vi "Configure Trace Statistics.vi"(7 "User Domain (0)":dbl, 8 "error in (no error)":errorcluster, 9 "Statistic Type (0: Peak to Peak)":i32(ring) items=["Peak to Peak", "Standard Deviation", "Mean", "Min", "Max"], 10 "Channel (1)":i32=1, 11 "VISA resource name":refnum<visa-resource-name>) -> (0 "error out":errorcluster, 3 "VISA resource name out":refnum<visa-resource-name>)   [LabVIEW 2018, in "Keysight PNA Series.lvlib"]
doc: "Configure Trace Statistics."
uses:
  Keysight PNA Series.lvlib
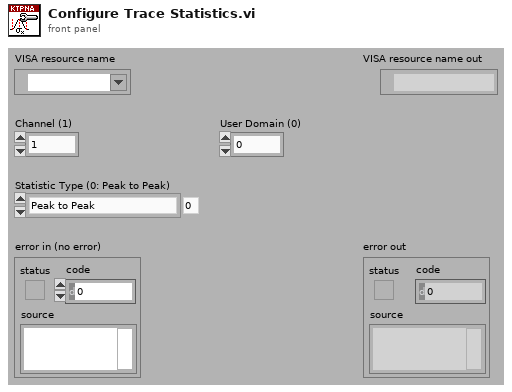
[diagram p1: front panel]
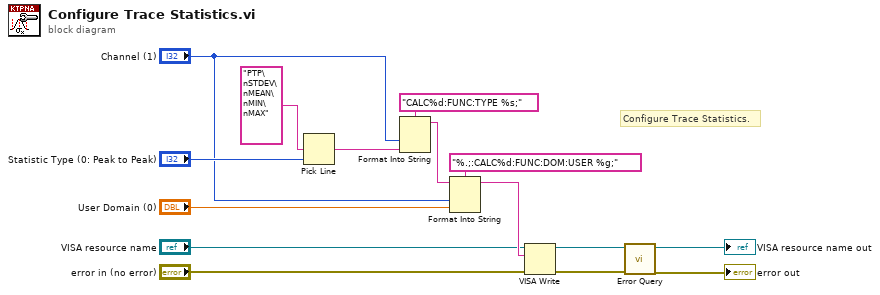
[diagram p0: block diagram]
diagram:
  # "Configure Trace Statistics."
  n1 = Pick Line(multi-line string="PTP\nSTDEV\nMEAN\nMIN\nMAX", line index="Statistic Type (0: Peak to Peak)") -> (output string=w11:string)  [unwired: 1 in]
  n2 = Format Into String(format string="CALC%d:FUNC:TYPE %s;", "Channel (1)", w11) -> (resulting string=w10:string)  [unwired: 2 in, 1 out]
  n3 = Format Into String(format string="%.;:CALC%d:FUNC:DOM:USER %g;", initial string=w10, "Channel (1)", "User Domain (0)") -> (resulting string=w7:string)  [unwired: 1 in, 1 out]
  n4 = VISA Write(VISA resource name="VISA resource name", write buffer=w7, error in (no error)="error in (no error)") -> (VISA resource name out=w4:refnum<visa-resource-name>, error out=w3:errorcluster)  [unwired: 1 out]
  n5 = call "Error Query.vi"("error in (no error)"=w3, "VISA resource name"=w4) -> ("error out"=→"error out":errorcluster, "VISA resource name out"=→"VISA resource name out":refnum<visa-resource-name>)  [unwired: 6 in, 2 out]
